vi "SUB_run_exeFile_NoWait.vi"(3 "exe filename":string) -> (0 "code":i32)   [LabVIEW 2011]
panel:
  out "stripped path":path
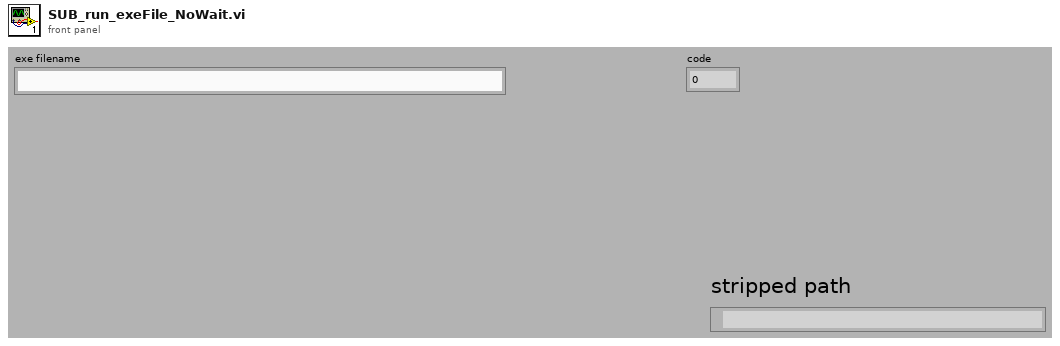
[diagram p1: front panel]
types:
  T1 = enum32{"invalid app kind", "Development System", "Run Time System", "Student Edition", "Embedded LabVIEW", "Evaluation", "Custom"}
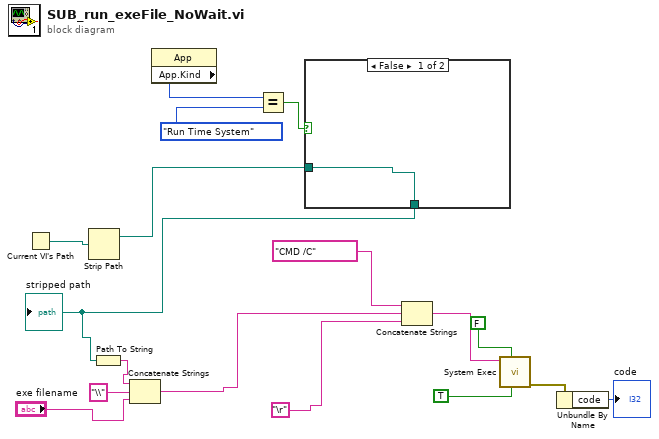
[diagram p0: block diagram]
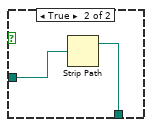
[diagram p2: hidden frame]
diagram:
  n1 = Current VI's Path() -> (path=w12:path)
  n2 = Strip Path(path=w12) -> (stripped path=w8:path)  [unwired: 1 out]
  n3 = property class="App"() -> ("App.Kind"=w9:T1)  [unwired: 2 in, 2 out]
  n4 = Equal?(x=w9, y=T1."Run Time System" ("Application:Kind")) -> (x = y?=w11:bool)
  n5 = case shown="False" w11 {
    tunnel: [w18 w20] -> w7
    tunnel: w8 -> [w18 w19]
    frame False {
    }
    frame True {
      n6 = Strip Path(path=w19) -> (stripped path=w20:path)  [unwired: 1 out]
    }
  }
  "stripped path" <- w7
  n7 = Path To String(path=w7) -> (string=w6:string)
  n8 = Concatenate Strings(w6, "\\", "exe filename") -> (w3:string)
  n9 = Concatenate Strings("CMD /C", w3, "\r") -> (w15:string)
  n10 = call <vilib>:"System Exec.vi"("run minimized? (F)"=TRUE, "wait until completion? (T)"=FALSE, "command line"=w15) -> ("error out"=w2:errorcluster)  [unwired: 5 in, 3 out]
  n11 = Unbundle By Name(w2) -> ("code"=→"code":i32)
